vi "Get Elevation.vi"(0 "GMaps API in":refnum<class "GMaps API.lvclass">, 5 "error in (no error)":errorcluster) -> (14 "GMaps API out":refnum<class "GMaps API.lvclass">, 15 "Elevation":cluster{"Elevation":string, "Resolution":string}, 19 "error out":errorcluster)   [LabVIEW 2016, in "GMaps API.lvclass"]
doc: "Gets elevation for all locations on the surface of the earth."
uses:
  GMaps API.lvclass
  GMaps API.lvclass/GMaps API.ctl
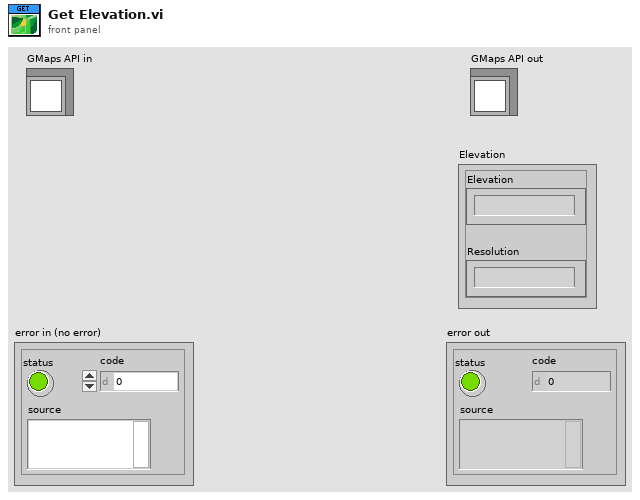
[diagram p1: front panel]
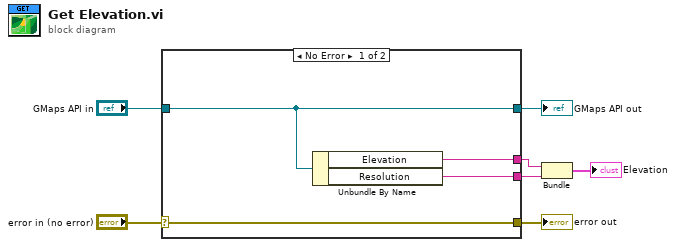
[diagram p0: block diagram]
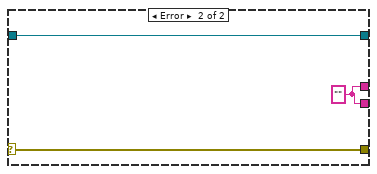
[diagram p2: hidden frame]
diagram:
  n1 = case shown="No Error" "error in (no error)" {
    selector: "error in (no error)" -> [w11 w14]
    tunnel: [w11 w14] -> w6
    tunnel: [w10 w13] -> w4
    tunnel: "GMaps API in" -> [w10 w13]
    tunnel: [w9 w12] -> w3
    tunnel: [w8 w12] -> w2
    frame No Error {
      n2 = Unbundle By Name(w10) -> ("Elevation"=w9:string, "Resolution"=w8:string)
    }
    frame Error {
      w12 = ""
    }
  }
  "error out" <- w6
  "GMaps API out" <- w4
  n3 = Bundle("Elevation"=w3, "Resolution"=w2) -> (→"Elevation":cluster{"Elevation":string, "Resolution":string})  [unwired: 1 in]
